vi "KE2182 Readout.vi"() -> ()   [LabVIEW 2018]
uses:
  Keithley 2182/Keithley 2182.lvlib
  KE2182 Voltage.vi
panel:
  in  "Integration Time (s)":dbl
  out "error out":errorcluster
  in  "?":bool
  out "KE2182 Voltage (V)":dbl
  in  "DC Voltmeter":refnum<visa-resource-name>
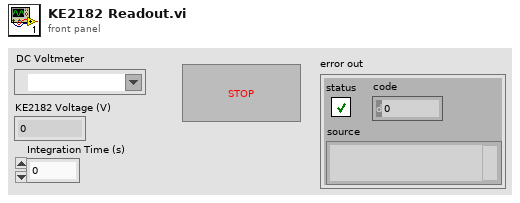
[diagram p1: front panel]
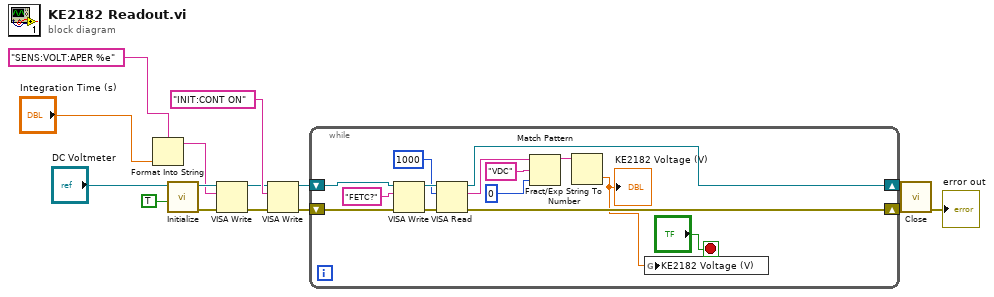
[diagram p0: block diagram]
diagram:
  n1 = Format Into String(format string="SENS:VOLT:APER %e" ("write buffer"), "Integration Time (s)") -> (resulting string=w1:string)  [unwired: 2 in, 1 out]
  n2 = call "Initialize.vi"("Reset (True)"=TRUE, "VISA resource name"="DC Voltmeter") -> ("error out"=w13:errorcluster, "VISA resource name out"=w12:refnum<visa-resource-name>)  [unwired: 8 in]
  n3 = VISA Write(VISA resource name=w12, write buffer=w1, error in (no error)=w13) -> (VISA resource name out=w7:refnum<visa-resource-name>, error out=w6:errorcluster)  [unwired: 1 out]
  n4 = VISA Write(VISA resource name=w7, write buffer="INIT:CONT ON", error in (no error)=w6) -> (VISA resource name out=w4:refnum<visa-resource-name>, error out=w5:errorcluster)  [unwired: 1 out]
  n5 = while {
    shift-right: [w19] -> w11
    shift-left: w4 -> [w29]
    shift-right: [w18] -> w10
    shift-left: w5 -> [w28]
    stop <- "?" stop-if-true
    n6 = VISA Write(VISA resource name=w29, write buffer="FETC?", error in (no error)=w28) -> (VISA resource name out=w27:refnum<visa-resource-name>, error out=w26:errorcluster)  [unwired: 1 out]
    n7 = VISA Read(VISA resource name=w27, byte count=u32 1000, error in (no error)=w26) -> (VISA resource name out=w19:refnum<visa-resource-name>, read buffer=w20:string, error out=w18:errorcluster)  [unwired: 1 out]
    n8 = Match Pattern(string=w20, regular expression="VDC", offset (0)=0) -> (before substring=w21:string)  [unwired: 3 out]
    n9 = Fract/Exp String To Number(string=w21) -> (number=w16:dbl)  [unwired: 3 in, 1 out]
    "KE2182 Voltage (V)" <- w16
    n10 = global write "KE2182 Voltage.vi" "KE2182 Voltage (V)"(w16) -> ()
  }
  n11 = call "Close.vi"("error in (no error)"=w10, "VISA resource name"=w11) -> ("error out"=→"error out":errorcluster)  [unwired: 9 in]
